vi "aux-conf-loader.vi"(11 "DIrectory (AUXI)":string="AUXI") -> (0 "error out":errorcluster, 3 "Array":T1[](array[typedef]) {"Period" format="Period [s]: %d"; "Pulse" format="Pulse [s]: %d"})   [LabVIEW 2024]
uses:
  controls/type.aux.ctl
  <vilib>/Utility/error.llb/Clear Errors.vi
  <vilib>/Utility/libraryn.llb/Create Directory Recursive.vi
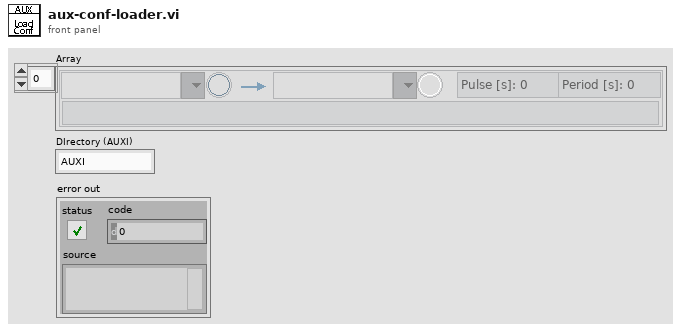
[diagram p1: front panel]
types:
  T1 = typedef "type.aux.ctl" = cluster{"Source":string, "SourceStatus":bool, "Dest":string, "DestStatus":bool, "Pulse":u16, "Period":u16, "Proc Name":string}
  T2 = typedef "UiStepBuilder.ctl" = cluster{"Step Function":T3, "ParamString":string, "Step Label":string}
  T3 = typedef "type.step-builder.ctl" = enum16{"NO_OPERATION", "DELAY-JUMP", "DELAY", "JUMP", "COMPLETE", "SCHEDULER", "IRR-CHECK", "UNIT-CHECK", "UNIT-SAMPLE", "UNIT-DOSE", "LOG-REPORT", "LOG-MESSAGE", "IO-READ", "IO-READ-MANY", "IO-WRITE", "IO-COMPARE-OUT", "IO-COMPARE-IN", "PROC-START", "PROC-STOP", "PROC-LOAD", "PROC-IS-COMPLETED", "RECORD-MOVE", "GET-RH", "GET-UV", "GET-WD", "GET-WS", "OCS-CHECK", "OCS-RECORD"}
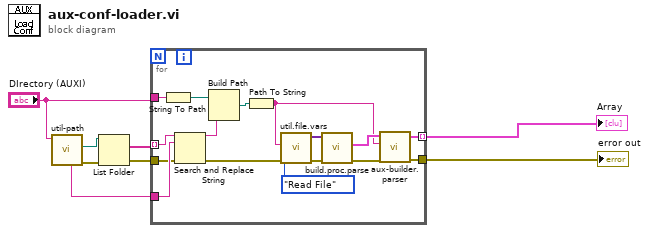
[diagram p0: block diagram]
diagram:
  n1 = call "util-path.vi"("append path (ie. folder\\filename.*)"="DIrectory (AUXI)") -> ("error out"=w3:errorcluster, "SelectedPath"=w7:path, ".extension (.prc)"=w6:string)  [unwired: 6 in, 2 out]
  n2 = List Folder(path=w7, error in=w3) -> (filenames=w2:string[], error out=w4:errorcluster)  [unwired: 2 in, 2 out]
  n3 = for {
    tunnel: w2 -> [w16] mode=indexing
    tunnel: [w21] -> w1 mode=indexing
    tunnel: w4 -> [w14]
    tunnel: [w18] -> w5
    tunnel: "DIrectory (AUXI)" -> [w17]
    tunnel: w6 -> [w15]
    n4 = String To Path(string=w17) -> (path=w10:path)
    n5 = Search and Replace String(input string=w16, search string=w15, error in=w14) -> (result string=w12:string, error out=w13:errorcluster)  [unwired: 5 in, 2 out]
    n6 = Build Path(base path=w10, name or relative path=w12) -> (appended path=w11:path)
    n7 = Path To String(path=w11) -> (string=w9:string)
    n8 = call "util.file.vars.vi"("Operation(Read)"=enum16{"Read File", "Write File"}."Read File", "error in"=w13, "Proc Name(open dialog if empty)"=w9) -> ("error out"=w20:errorcluster, "Vars[] out"=w23:variant[])  [unwired: 4 in, 3 out]
    n9 = call "build.proc.parse.vi"("error"=w20, "Array in"=w23) -> ("error out"=w19:errorcluster, "Flow Steps"=w22:T2[])  [unwired: 7 in, 1 out]
    n10 = call "aux-builder.parser.vi"("error in"=w19, "Proc Name"=w9, "Flow"=w22) -> ("error out"=w18:errorcluster, "Aux Conf out"=w21:T1)  [unwired: 7 in]
  }
  "error out" <- w5
  "Array" <- w1
